vi "Read Settings Cluster.vi"(8 "error in":errorcluster, 10 "variant":variant, 11 "Name":string) -> (0 "error out":errorcluster, 2 "Devicetype Variable \nData":string[][](array[string]))   [LabVIEW 2013]
doc: "This vi Read Settings cluster and update or add deviectype variable in Database for specified Device.\n\nInput\n1. Settings cluster\n2. DeviceName\n3. Error in\n\nOutput\n1. Devicetype Variable List\n2. Error Out"
uses:
  Device Drivers/shared/numericVariable_TypeDef.ctl
  Device Drivers/BaseDriver/BaseDriver.lvclass
panel:
  out "Data Name":string
  out "Array of VData":variant[](array[variant])
  # "(Taken for nested cluster names\neg Target cluster having x and y element \nthen name should be Target.X and Target.y)"
  # "Read variant input and parse Devicetype variable information from variant"
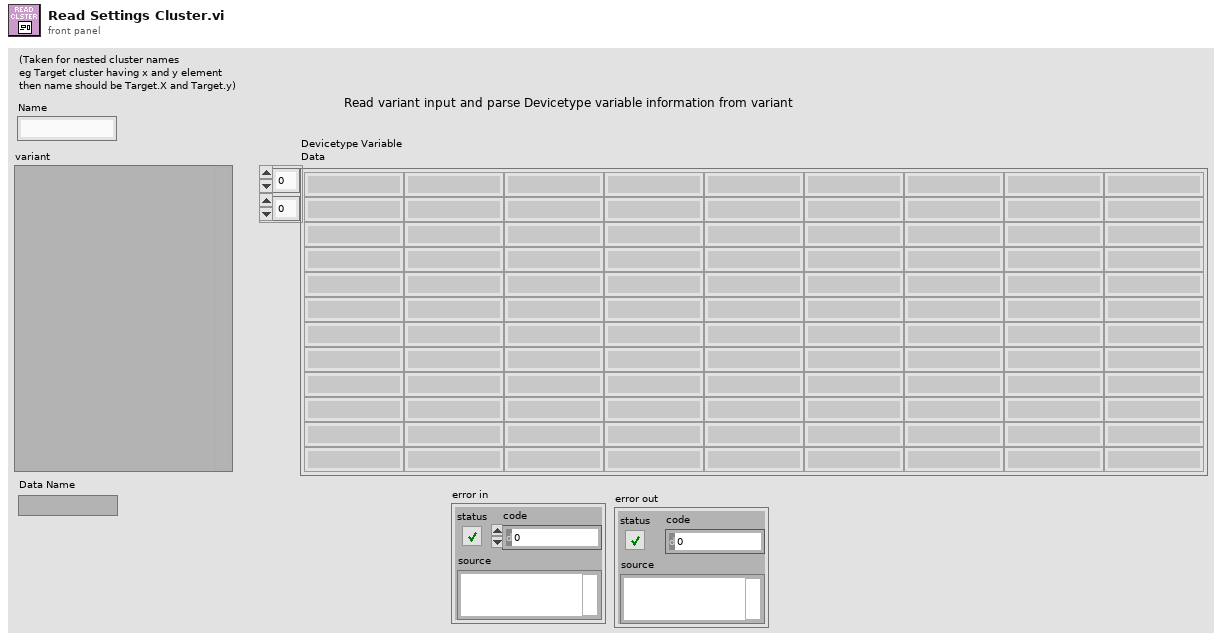
[diagram p1: front panel]
types:
  T1 = typedef "BaseDriver.lvclass/numericVariable_TypeDef.ctl" = cluster{"Value":dbl, "Min":dbl, "Max":dbl, "StepSize":dbl, "Tolerance":dbl, "ValueActual":dbl}
  T2 = cluster{"name":string, "value":string, "min":string, "max":string, "stepsize":string, "units":string, "variabletype":string, "tolerance":string, "valueactual":string}
  T3 = typedef "Type Descriptor Header__ogtk.ctl" = cluster{"length":u16, "private":u8, "type":T4, "# elements":u16}
  T4 = typedef "Type Descriptor Enumeration__ogtk.ctl" = enum8{"<Null>", "I8", "I16", "I32", "I64", "U8", "U16", "U32", "U64", "SGL", "DBL", "EXT", "CSG", "CDB", "CXT", "0x0F", "0x10", "0x11", "0x12", "0x13", "0x14", "Enum U8", "Enum U16", "Enum U32", "Enum U64", "SGL PQ", "DBL PQ", "EXT PQ", "CSG PQ", "CDB PQ", "CXT PQ", "0x1F", "0x20", "Boolean", "0x22", "0x23", "0x24", "0x25", "0x26", "0x27", "0x28", "0x29", "0x2A", "0x2B", "0x2C", "0x2D", "0x2E", "0x2F", "String", "0x31", "Path", "Pict", "0x34", "0x35", "0x36", "DAQ", "0x38", "0x39", "0x3A", "0x3B", "0x3C", "0x3D", "0x3E", "0x3F", "Array", "0x41", "0x42", "0x43", "0x44", "0x45", "0x46", "0x47", "0x48", "0x49", "0x4A", "0x4B", "0x4C", "0x4D", "0x4E", "0x4F", "Cluster", "0x51", "0x52", "Variant", "Waveform", "0x55", "0x56", "0x57", "0x58", "0x59", "0x5A", "0x5B", "0x5C", "0x5D", "0x5E", "0x5F", "0x60", "0x61", "0x62", "0x63", "0x64", "0x65", "0x66", "0x67", "0x68", "0x69", "0x6A", "0x6B", "0x6C", "0x6D", "0x6E", "0x6F", "Refnum"}
  T5 = typedef "Type Descriptor__ogtk.ctl" = i16[]
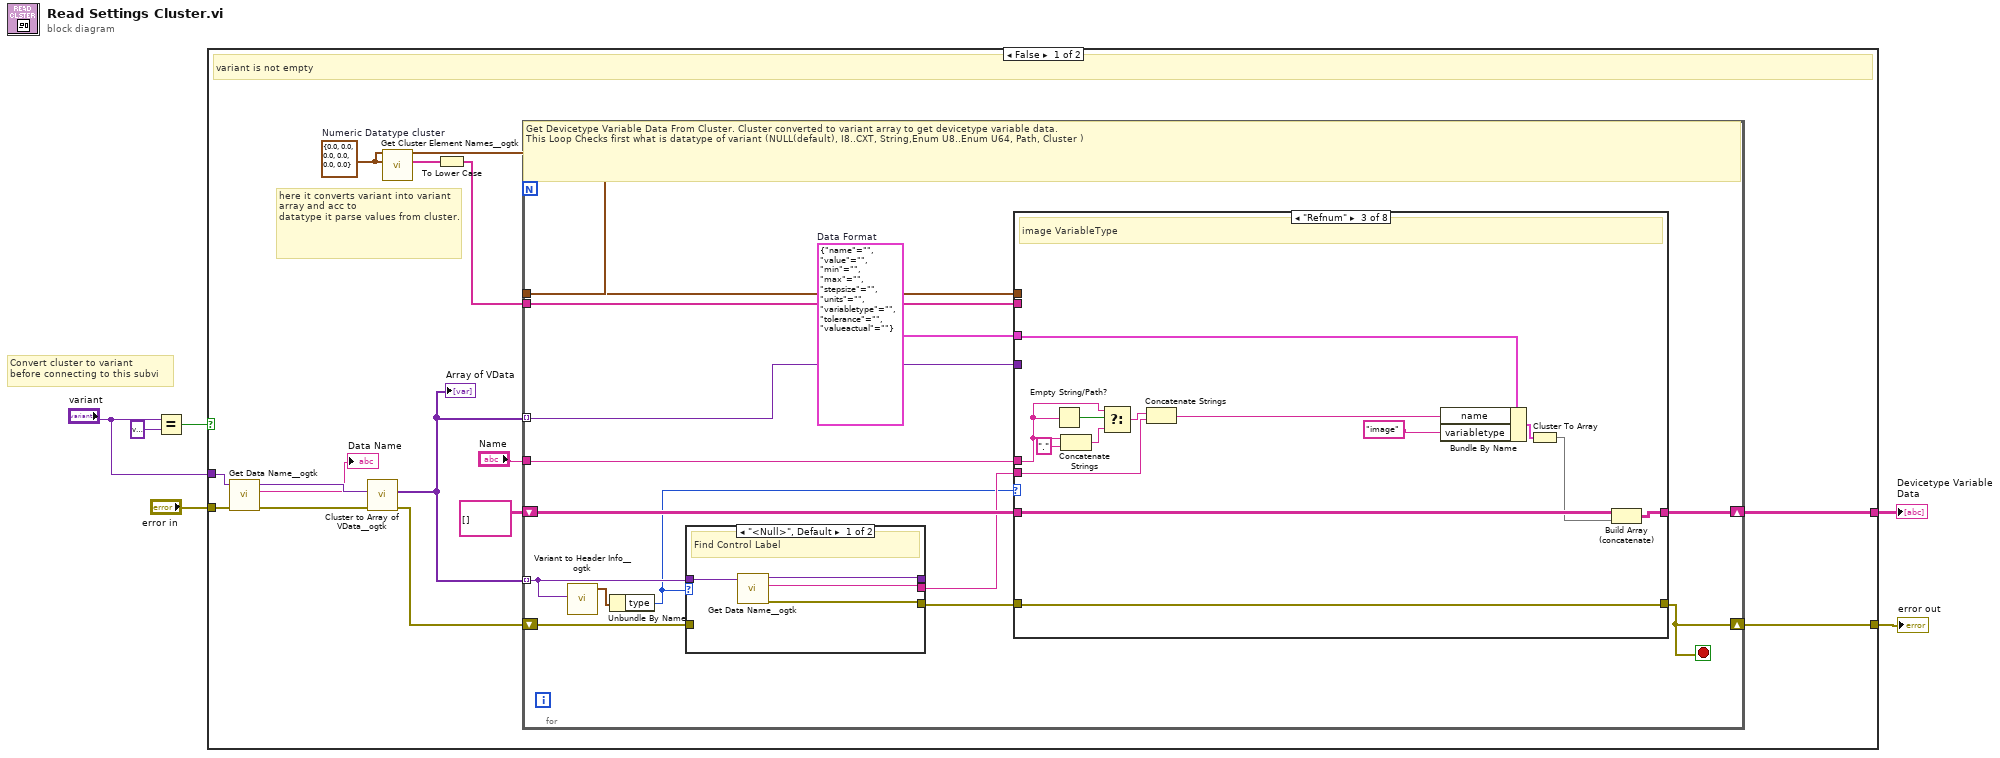
[diagram p0: block diagram]
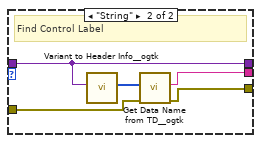
[diagram p2: hidden frame]
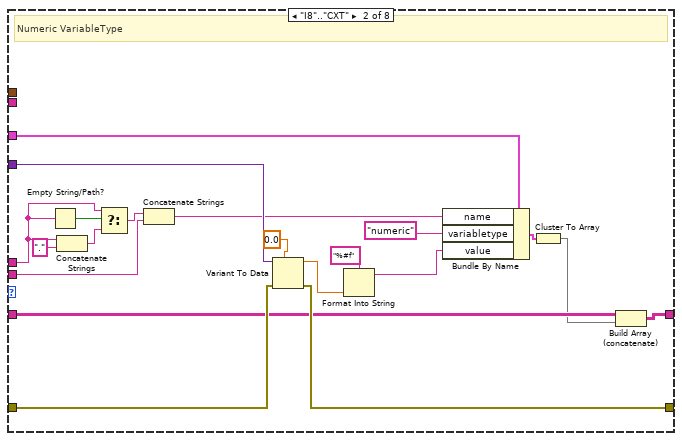
[diagram p4: hidden frame]
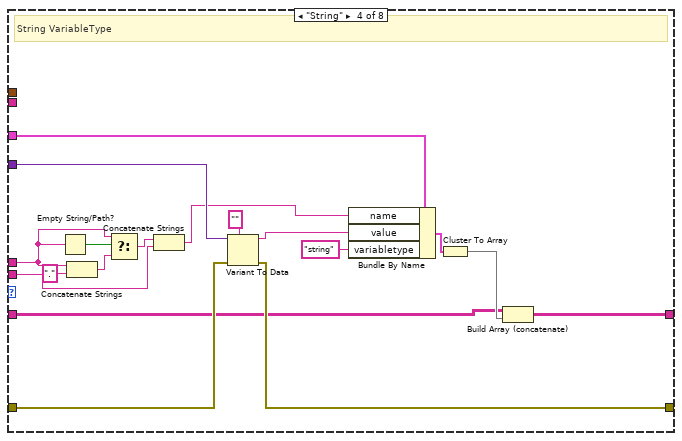
[diagram p5: hidden frame]
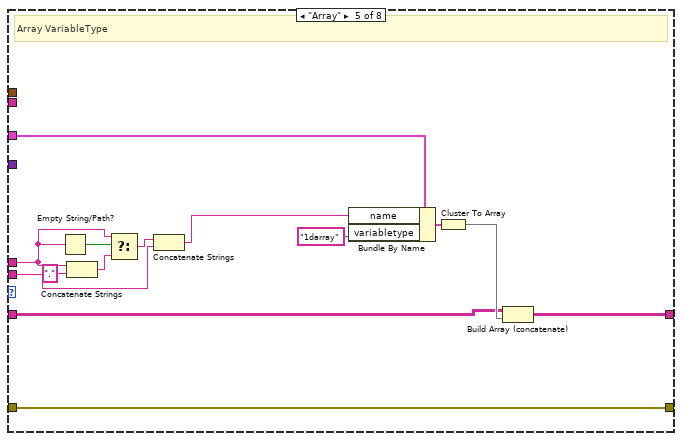
[diagram p6: hidden frame]
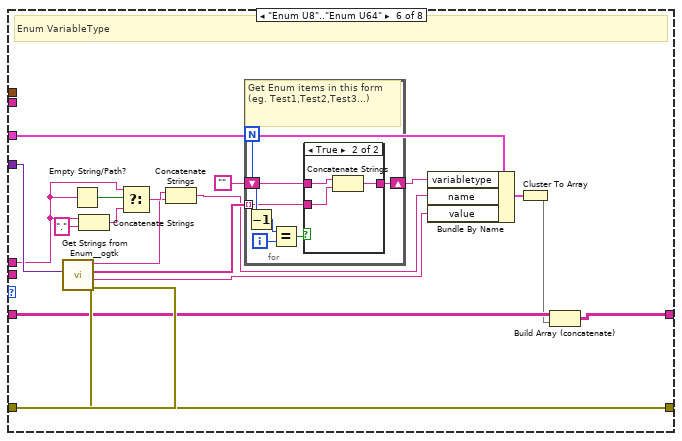
[diagram p7: hidden frame]
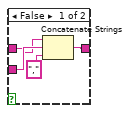
[diagram p8: hidden frame]
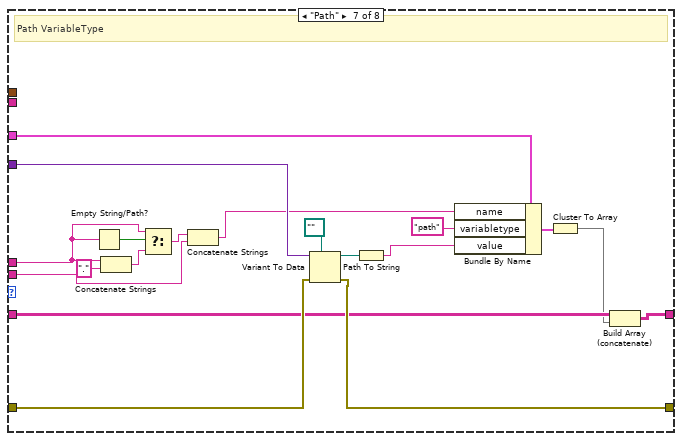
[diagram p9: hidden frame]
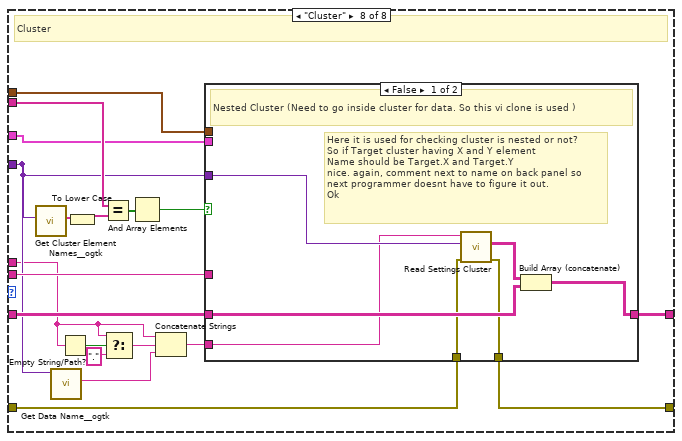
[diagram p10: hidden frame]
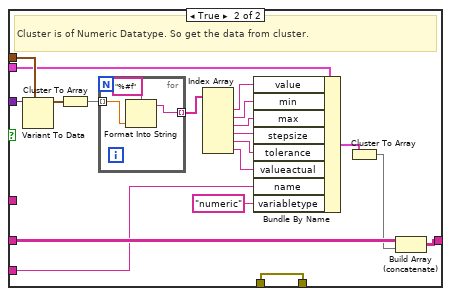
[diagram p11: hidden frame]
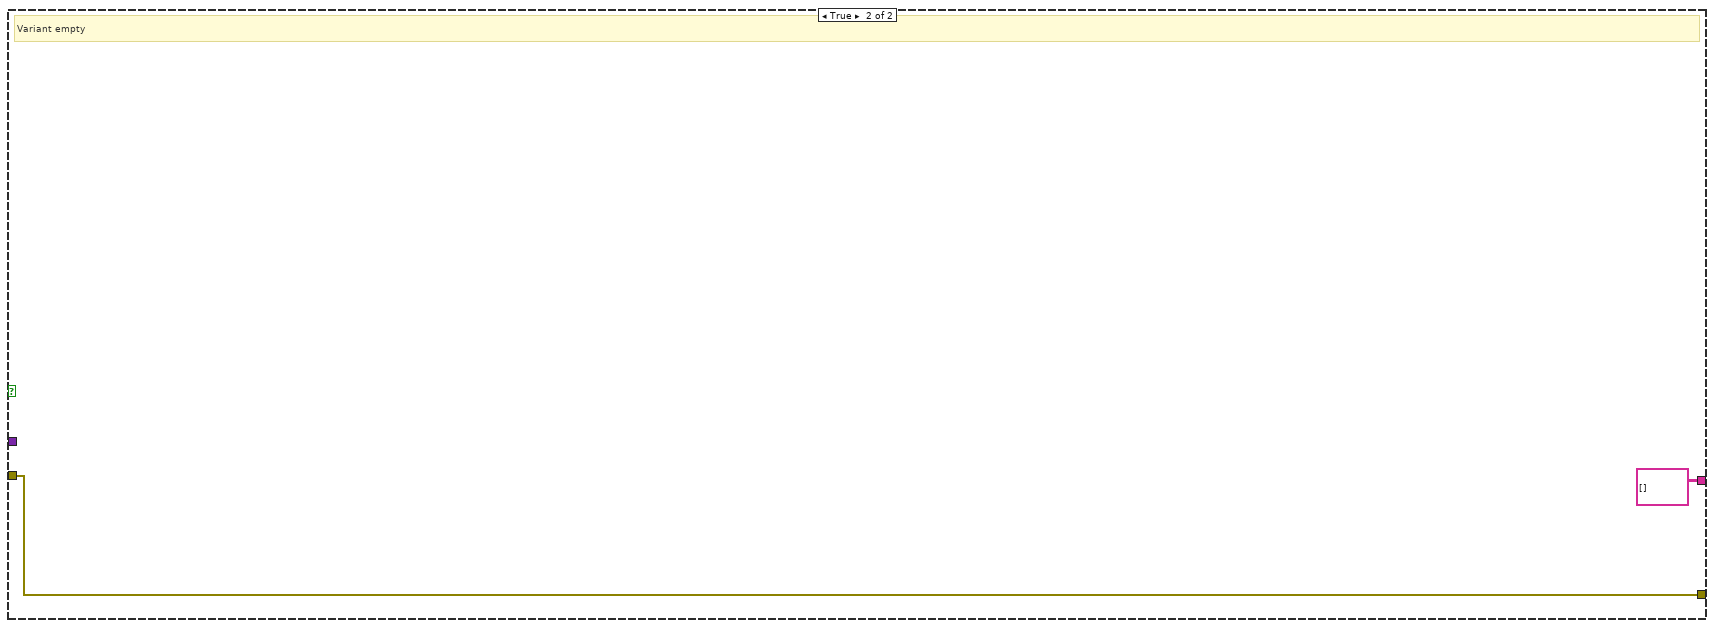
[diagram p12: hidden frame]
diagram:
  # "Convert cluster to variant \nbefore connecting to this subvi"
  n1 = Equal?(x="variant", y=variant) -> (x = y?=w4:bool)
  n2 = case shown="False" w4 {
    tunnel: "error in" -> [w16 w212]
    tunnel: "variant" -> [w9 _]
    tunnel: [w8 string[][] []] -> w2
    tunnel: [w7 w212] -> w1
    frame False {
      w11 = T1 {"Value"=0.0, "Min"=0.0, "Max"=0.0, "StepSize"=0.0, "Tolerance"=0.0, "ValueActual"=0.0}  # Numeric Datatype cluster
      # "here it converts variant into variant array and acc to \ndatatype it parse values from cluster."
      # "variant is not empty"
      n3 = call "Get Data Name__ogtk.vi"("error in (no error)"=w16, "Data"=w9) -> ("error out"=w18:errorcluster, "Data Name"=→"Data Name":string, "Data dup"=w20:variant)  [unwired: 7 in]
      n4 = call "Cluster to Array of VData__ogtk.vi"("error in (no error)"=w18, "Cluster"=w20) -> ("error out"=w17:errorcluster, "Array of VData"=w15:variant[])  [unwired: 8 in]
      "Array of VData" <- w15
      n5 = call "Get Cluster Element Names__ogtk.vi"("Cluster"=w11) -> ("Element Names"=w12:string[])  [unwired: 9 in, 1 out]
      n6 = To Lower Case(string=w12) -> (all lower case string=w10:string[])
      n7 = for {
        tunnel: w15 -> [w32] mode=indexing
        shift-right: [w33] -> w8
        shift-left: string[][] [] -> [w34]
        shift-right: [w23] -> w7
        shift-left: w17 -> [w31]
        tunnel: w15 -> [w25] mode=indexing
        tunnel: "Name" -> [w24]
        tunnel: w11 -> [w22]
        tunnel: w10 -> [w21]
        stop <- w23 stop-if-true
        w26 = T2 {"name"="", "value"="", "min"="", "max"="", "stepsize"="", "units"="", "variabletype"="", "tolerance"="", "valueactual"=""}  # Data Format
        # "Get Devicetype Variable Data From Cluster. Cluster converted to variant array to get devicetype variable data.\nThis Loop Checks first what is datatype of variant (NULL(default), I8..CXT, String,Enum U8..Enum U64, Path, Cluster )"
        n8 = call "Variant to Header Info__ogtk.vi"("Variant"=w32) -> ("Type Descriptor Header"=w27:T3)  [unwired: 3 in, 2 out]
        n9 = Unbundle By Name(w27) -> ("type"=w28:T4)
        n10 = case shown="\"<Null>\", Default" w28 {
          tunnel: w31 -> [_ w43]
          tunnel: [w37 w42] -> w30
          tunnel: w32 -> [w38 w39]
          tunnel: [w36 w40] -> w29
          tunnel: [w35 w39] -> _
          frame "<Null>", Default {
            # "Find Control Label"
            n11 = call "Get Data Name__ogtk.vi"("Data"=w38) -> ("error out"=w37:errorcluster, "Data Name"=w36:string, "Data dup"=w35:variant)  [unwired: 8 in]
          }
          frame "String" {
            # "Find Control Label"
            n12 = call "Variant to Header Info__ogtk.vi"("Variant"=w39) -> ("Type Descriptor"=w41:T5)  [unwired: 3 in, 2 out]
            n13 = call "Get Data Name from TD__ogtk.vi"("error in (no error)"=w43, "Type Descriptor"=w41) -> ("error"=w42:errorcluster, "name"=w40:string)  [unwired: 8 in]
          }
        }
        n14 = case shown="\"Refnum\"" w28 {
          tunnel: w25 -> [_ w62 _ w97 _ w130 w160 w172]
          tunnel: w21 -> [_ _ _ _ _ _ _ w179]
          tunnel: w30 -> [w44 w60 w66 w93 w98 w129 w159 w164]
          tunnel: [w44 w59 w66 w91 w98 w128 w158 w165] -> w23
          tunnel: w34 -> [w45 w55 w76 w88 w107 w121 w154 w174]
          tunnel: [w45 w53 w74 w87 w106 w119 w152 w173] -> w33
          tunnel: w29 -> [_ w46 w67 w80 w99 _ w145 w175]
          tunnel: w26 -> [_ w65 w79 w95 w111 w125 w161 w176]
          tunnel: w22 -> [_ _ _ _ _ _ _ w177]
          tunnel: w24 -> [_ w50 w71 w83 w102 w115 w148 w167]
          frame "<Null>", Default {
            # "NULL"
          }
          frame "I8".."CXT" {
            # "Numeric VariableType"
            n15 = Empty String/Path?(string/path=w50) -> (empty?=w52:bool)
            n16 = Concatenate Strings(w50, "." ("string")) -> (w51:string)
            n17 = Select(t=w50, s=w52, f=w51) -> (s? t:f=w47:string)
            n18 = Concatenate Strings(w47, w46) -> (w48:string)
            n19 = Variant To Data(error in=w60, type=0.0, Variant=w62) -> (data=w57:dbl, error out=w59:errorcluster)
            n20 = Format Into String(format string="%#f", w57) -> (resulting string=w56:string)  [unwired: 2 in, 1 out]
            n21 = Bundle By Name(cluster=w65, "name"=w48, "variabletype"="numeric", "value"=w56) -> (w63:T2)
            n22 = Cluster To Array(cluster=w63) -> (array=w54:string[])
            n23 = Build Array (concatenate)(w55, w54) -> (w53:string[][])
          }
          frame "Refnum" {
            # "image VariableType"
            n24 = Empty String/Path?(string/path=w71) -> (empty?=w73:bool)
            n25 = Concatenate Strings(w71, "." ("string")) -> (w72:string)
            n26 = Select(t=w71, s=w73, f=w72) -> (s? t:f=w68:string)
            n27 = Concatenate Strings(w68, w67) -> (w69:string)
            n28 = Bundle By Name(cluster=w79, "name"=w69, "variabletype"="image") -> (w77:T2)
            n29 = Cluster To Array(cluster=w77) -> (array=w75:string[])
            n30 = Build Array (concatenate)(w76, w75) -> (w74:string[][])
          }
          frame "String" {
            # "String VariableType"
            n31 = Empty String/Path?(string/path=w83) -> (empty?=w86:bool)
            n32 = Concatenate Strings(w83, "." ("string")) -> (w85:string)
            n33 = Select(t=w83, s=w86, f=w85) -> (s? t:f=w81:string)
            n34 = Concatenate Strings(w81, w80) -> (w82:string)
            n35 = Variant To Data(error in=w93, type="", Variant=w97) -> (data=w92:string, error out=w91:errorcluster)
            n36 = Bundle By Name(cluster=w95, "name"=w82, "value"=w92, "variabletype"="string") -> (w94:T2)
            n37 = Cluster To Array(cluster=w94) -> (array=w89:string[])
            n38 = Build Array (concatenate)(w88, w89) -> (w87:string[][])
          }
          frame "Array" {
            # "Array VariableType"
            n39 = Empty String/Path?(string/path=w102) -> (empty?=w105:bool)
            n40 = Concatenate Strings(w102, "." ("string")) -> (w104:string)
            n41 = Select(t=w102, s=w105, f=w104) -> (s? t:f=w100:string)
            n42 = Concatenate Strings(w100, w99) -> (w101:string)
            n43 = Bundle By Name(cluster=w111, "name"=w101, "variabletype"="1darray") -> (w110:T2)
            n44 = Cluster To Array(cluster=w110) -> (array=w108:string[])
            n45 = Build Array (concatenate)(w107, w108) -> (w106:string[][])
          }
          frame "Enum U8".."Enum U64" {
            # "Enum VariableType"
            n46 = call "Get Strings from Enum__ogtk.vi"("error in (no error)"=w129, "Enum"=w130) -> ("error out"=w128:errorcluster, "String Value"=w123:string, "Enum Strings"=w127:string[], "Enum Name"=w112:string)  [unwired: 6 in]
            n47 = Empty String/Path?(string/path=w115) -> (empty?=w118:bool)
            n48 = Concatenate Strings(w115, "." ("string")) -> (w117:string)
            n49 = Select(t=w115, s=w118, f=w117) -> (s? t:f=w113:string)
            n50 = Concatenate Strings(w113, w112) -> (w114:string)
            n51 = for {
              N -> [w137]
              tunnel: w127 -> [w132] mode=indexing
              shift-right: [w133] -> w124
              shift-left: "" -> [w131]
              i -> [w135]
              # "Get Enum items in this form (eg. Test1,Test2,Test3...)"
              n52 = Decrement(x=w137) -> (x-1=w136:i32)
              n53 = Equal?(x=w136, y=w135) -> (x = y?=w134:bool)
              n54 = case shown="True" w134 {
                tunnel: w132 -> [w140 w143]
                tunnel: [w139 w142] -> w133
                tunnel: w131 -> [w138 w144]
                frame False {
                  n55 = Concatenate Strings(w138, w140, ",") -> (w139:string)
                }
                frame True {
                  n56 = Concatenate Strings(w144, w143) -> (w142:string)
                }
              }
            }
            n57 = Bundle By Name(cluster=w125, "variabletype"=w124, "name"=w114, "value"=w123) -> (w122:T2)
            n58 = Cluster To Array(cluster=w122) -> (array=w120:string[])
            n59 = Build Array (concatenate)(w121, w120) -> (w119:string[][])
          }
          frame "Path" {
            # "Path VariableType"
            n60 = Empty String/Path?(string/path=w148) -> (empty?=w151:bool)
            n61 = Concatenate Strings(w148, "." ("string")) -> (w150:string)
            n62 = Select(t=w148, s=w151, f=w150) -> (s? t:f=w146:string)
            n63 = Concatenate Strings(w146, w145) -> (w147:string)
            n64 = Variant To Data(error in=w159, type=path "", Variant=w160) -> (data=w156:path, error out=w158:errorcluster)
            n65 = Path To String(path=w156) -> (string=w155:string)
            n66 = Bundle By Name(cluster=w161, "name"=w147, "variabletype"="path", "value"=w155) -> (w162:T2)
            n67 = Cluster To Array(cluster=w162) -> (array=w153:string[])
            n68 = Build Array (concatenate)(w154, w153) -> (w152:string[][])
          }
          frame "Cluster" {
            # "Cluster"
            n69 = call "Get Cluster Element Names__ogtk.vi"("Cluster"=w172) -> ("Element Names"=w182:string[])  [unwired: 9 in, 1 out]
            n70 = call "Get Data Name__ogtk.vi"("Data"=w172) -> ("Data Name"=w168:string)  [unwired: 8 in, 2 out]
            n71 = Empty String/Path?(string/path=w167) -> (empty?=w169:bool)
            n72 = To Lower Case(string=w182) -> (all lower case string=w181:string[])
            n73 = Equal?(x=w179, y=w181) -> (x = y?=w180:bool[])
            n74 = Select(t=w167, s=w169, f="." ("string")) -> (s? t:f=w171:string)
            n75 = And Array Elements(Boolean array=w180) -> (logical AND=w178:bool)
            n76 = Concatenate Strings(w167, w171, w168) -> (w166:string)
            n77 = case shown="False" w178 {
              tunnel: w177 -> [_ w206]
              tunnel: w172 -> [w189 w208]
              tunnel: w176 -> [_ w205]
              tunnel: w175 -> [_ _]
              tunnel: w174 -> [w188 w194]
              tunnel: [w187 w192] -> w173
              tunnel: w166 -> [w185 w191]
              tunnel: w164 -> [w184 w190]
              tunnel: [w183 w190] -> w165
              frame False {
                # "Here it is used for checking cluster is nested or not?\nSo if Target cluster having X and Y element \nName should be Target.X and Target.Y\nnice. again, comment next to name on back panel so\nnext programmer doesnt have to figure it out.\nOk"
                # "Nested Cluster (Need to go inside cluster for data. So this vi clone is used )"
                n78 = call "Read Settings Cluster.vi"("error in"=w184, "variant"=w189, "Name"=w185) -> ("error out"=w183:errorcluster, "Devicetype Variable \nData"=w186:string[][])  [unwired: 7 in]
                n79 = Build Array (concatenate)(w186, w188) -> (w187:string[][])
              }
              frame True {
                # "Cluster is of Numeric Datatype. So get the data from cluster."
                n80 = Variant To Data(type=w206, Variant=w208) -> (data=w196:T1)  [unwired: 1 in, 1 out]
                n81 = Cluster To Array(cluster=w196) -> (array=w207:dbl[])
                n82 = for {
                  tunnel: w207 -> [w211] mode=indexing
                  tunnel: [w210] -> w204 mode=indexing
                  n83 = Format Into String(format string="%#f", w211) -> (resulting string=w210:string)  [unwired: 2 in, 1 out]
                }
                n84 = Index Array(array=w204) -> (element #1=w203:string, element #2=w202:string, element #3=w201:string, element #4=w200:string, element #5=w199:string, element #6=w198:string)  [unwired: 6 in]
                n85 = Bundle By Name(cluster=w205, "value"=w203, "min"=w202, "max"=w201, "stepsize"=w200, "tolerance"=w199, "valueactual"=w198, "name"=w191, "variabletype"="numeric") -> (w195:T2)
                n86 = Cluster To Array(cluster=w195) -> (array=w193:string[])
                n87 = Build Array (concatenate)(w194, w193) -> (w192:string[][])
              }
            }
          }
        }
      }
    }
    frame True {
      # "Variant empty"
    }
  }
  "error out" <- w1
  "Devicetype Variable \nData" <- w2
